vi "Xsquared Driver Control.vi"(10 "joystick input":dbl) -> (2 "out":dbl)   [LabVIEW 2012]
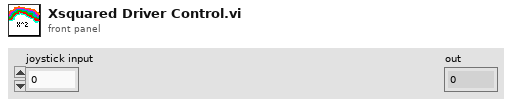
[diagram p1: front panel]
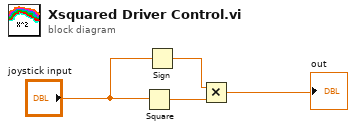
[diagram p0: block diagram]
diagram:
  n1 = Square(x="joystick input") -> (x^2=w2:dbl)
  n2 = Sign(1:"joystick input") -> (0:w3:dbl)
  n3 = Multiply(x=w3, y=w2) -> (x*y=→"out":dbl)
